vi "Initialize.vi"(7 "Channel Name":string="Setpoint.ch%d.SP", 8 "error in":errorcluster, 9 "Number of Channels":u32=1, 10 "Instance Name":string, 11 "Error Channels in":refnum<class "Error Channels.lvclass">) -> (0 "error out":errorcluster, 3 "Error Channels out":refnum<class "Error Channels.lvclass">)   [LabVIEW 2023, in "Error Channels.lvclass"]
uses:
  Error Channels.lvclass
  Error Channels.lvclass/Error Channels.ctl
  Utilities/Utilities.lvlib
  <vilib>/ADAS Replay HIL/Channels/Tag Wrapper/Tag Wrapper.lvlib
  <vilib>/ADAS Replay HIL/Channels/Tag Wrapper/Polymorphic/Set Default Value (I32).vi
  <vilib>/ADAS Replay HIL/Channels/Tag Wrapper/Polymorphic/Open Producer Tag (I32).vi
  <vilib>/ADAS Replay HIL/Channels/Tag Wrapper/Polymorphic/Open Consumer Tag (Boolean).vi
  <vilib>/ADAS Replay HIL/Channels/Tag Wrapper/Polymorphic/Set Default Value (Boolean).vi
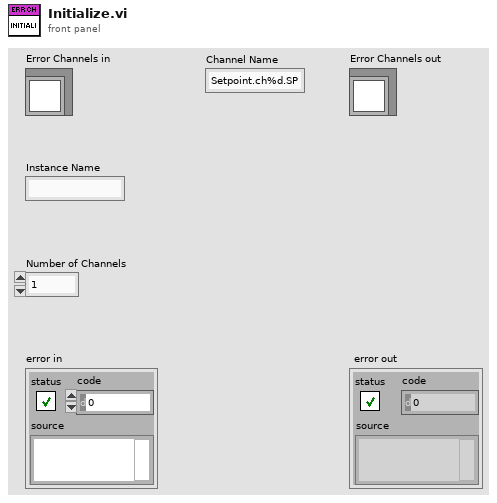
[diagram p1: front panel]
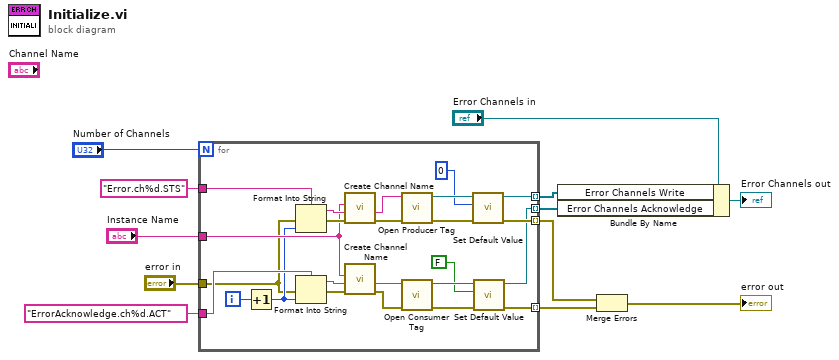
[diagram p0: block diagram]
diagram:
  n1 = for {
    N: "Number of Channels" -> [_]
    tunnel: [w31] -> w10 mode=indexing
    tunnel: "Error.ch%d.STS" ("ChannelName") -> [w27]
    tunnel: "Instance Name" -> [w18]
    tunnel: "error in" -> [w13]
    tunnel: [w21] -> w2 mode=indexing
    tunnel: "ErrorAcknowledge.ch%d.ACT" ("ChannelName") -> [w17]
    tunnel: [w15] -> w3 mode=indexing
    tunnel: [w14] -> w1 mode=indexing
    i -> [w29]
    n2 = Increment(x=w29) -> (x+1=w16:i32)
    n3 = Format Into String(format string=w27, error in=w13, w16) -> (resulting string=w32:string, error out=w30:errorcluster)  [unwired: 1 in]
    n4 = Format Into String(format string=w17, error in=w13, w16) -> (resulting string=w19:string, error out=w20:errorcluster)  [unwired: 1 in]
    n5 = call "Create Channel Name.vi"("error in"=w30, "Channel Name"=w32, "Plugin Name"=w18) -> ("error out"=w35:errorcluster, "Data Channel Name"=w33:string)  [unwired: 7 in]
    n6 = call "Create Channel Name.vi"("error in"=w20, "Channel Name"=w19, "Plugin Name"=w18) -> ("error out"=w24:errorcluster, "Data Channel Name"=w25:string)  [unwired: 7 in]
    n7 = call-poly <vilib>:"Open Producer Tag.vi"("error in"=w35, "Channel Name"=w33) -> ("error out"=w34:errorcluster, "ADAS HIL Channel"=w36:refnum<k21>)  [unwired: 8 in]
    n8 = call-poly <vilib>:"Open Consumer Tag.vi"("error in"=w24, "Channel Name"=w25) -> ("error out"=w23:errorcluster, "ADAS HIL Channel"=w26:refnum<k21>)  [unwired: 8 in]
    n9 = call-poly <vilib>:"Set Default Value.vi"("error in"=w34, "Default Value"=0, "ADAS HIL Channel in"=w36) -> ("error out"=w15:errorcluster, "ADAS HIL Channel out"=w31:refnum<k21>)  [unwired: 7 in]
    n10 = call-poly <vilib>:"Set Default Value.vi"("error in"=w23, "Default Value"=FALSE, "ADAS HIL Channel in"=w26) -> ("error out"=w21:errorcluster, "ADAS HIL Channel out"=w14:refnum<k21>)  [unwired: 7 in]
  }
  n11 = Bundle By Name(cluster="Error Channels in", "Error Channels Write"=w10, "Error Channels Acknowledge"=w1) -> (→"Error Channels out":refnum<class "Error Channels.lvclass">)
  n12 = Merge Errors(w3, w2) -> (→"error out":errorcluster)
